vi "Ej 4 Excel_1.vi"   [LabVIEW 2020]
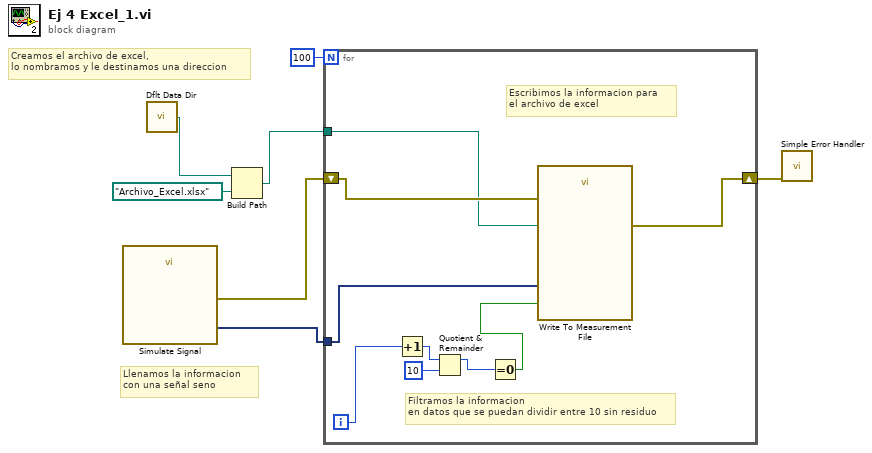
[diagram p0: block diagram]
diagram:
  # "Llenamos la informacion \ncon una señal seno"
  # "Creamos el archivo de excel,\nlo nombramos y le destinamos una direccion"
  n1 = call "Simulate Signal"() -> ("Sine"=w7:dynamicdata, "error out"=w5:errorcluster)  [unwired: 14 in]
  n2 = call <vilib>:"Dflt Data Dir.vi"() -> ("App:Default Data Directory"=w2:path)
  n3 = Build Path(base path=w2, name or relative path=path "Archivo_Excel.xlsx") -> (appended path=w1:path)
  n4 = for {
    N: 100 -> [_]
    tunnel: w7 -> [w16]
    shift-right: [w14] -> w4
    shift-left: w5 -> [w15]
    tunnel: w1 -> [w13]
    i -> [w11]
    # "Filtramos la informacion \nen datos que se puedan dividir entre 10 sin residuo"
    # "Escribimos la informacion para \nel archivo de excel"
    n5 = Increment(x=w11) -> (x+1=w12:i32)
    n6 = Quotient & Remainder(x=w12, y=10) -> (x-y*floor(x/y)=w9:i32)  [unwired: 1 out]
    n7 = Equal To 0?(x=w9) -> (x = 0?=w8:bool)
    n8 = call "Write To Measurement File"("Signals"=w16, "Flush? (T)"=w8, "error in (no error)"=w15, "Filename"=w13) -> ("error out"=w14:errorcluster)  [unwired: 13 in, 2 out]
  }
  n9 = call <vilib>:"Simple Error Handler.vi"("error in (no error)"=w4) -> ()  [unwired: 4 in, 5 out]
